vi "Read Size.vi"(11 "Product In":refnum<class "Product.lvclass">) -> (2 "Size":T1, 3 "Product Out":refnum<class "Product.lvclass">)   [LabVIEW 2018, in "Product.lvclass"]
uses:
  Product.lvclass
  Size.ctl
  Product.lvclass/Product.ctl
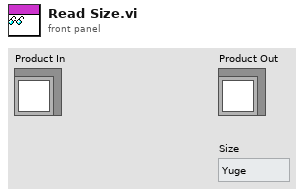
[diagram p1: front panel]
types:
  T1 = typedef "Product.lvclass/Size.ctl" = enum16{"Yuge", "Big", "Medium", "Small"}
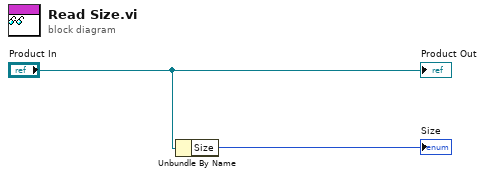
[diagram p0: block diagram]
diagram:
  n1 = Unbundle By Name("Product In") -> ("Size"=→"Size":T1)
  "Product Out" <- "Product In"
